vi "FL compute rule weights.vi"(7 "max num consequent membership fcns":i32, 8 "rule-invoked array":bool[](array[boolean]), 9 "output membership factors (u)":dbl[][](array[numeric]), 10 "input membership factors (u)":dbl[][](array[numeric]), 11 "fuzzy system in":T1 {"user MF interpolating polynomials"."coa_x(y) coeff" format="%.4g"; "user MF interpolating polynomials"."Area(y) coeff" format="%.4g"; "user MF interpolating polynomials"."X(y) coeff" format="%.4g"; "user MF interpolating polynomials"."Y(x) coeff" format="%.4g"; "user MF interpolating polynomials"."Y" format="%.4g"; "user MF interpolating polynomials"."X" format="%.4g"; "defuzzification method" items=["Center of Area", "Modified Center of Area", "Center of Sums", "Center of Maximum", "Mean of Maximum"]; "rules"."consequents"."Var Index" min=0; "rules"."consequents"."Cond" items=["=", "!="]; "rules"."consequents"."MF Index" min=0; "rules"."antecedents"."Var Index" min=0; "rules"."antecedents"."Cond" items=["=", "!="]; "rules"."antecedents"."MF Index" min=0; "rules"."consequent implication" items=["Minimum", "Product"]; "rules"."antecedent connective" items=["AND (Minimum)", "AND (Product)", "OR (Maximum)", "OR (Probabilistic)"]; "output variables"."MFs"."shape" items=["Triangle", "Trapezoid", "Singleton", "Sigmoid", "Gaussian", "User-Defined"]; "input variables"."MFs"."shape" items=["Triangle", "Trapezoid", "Singleton", "Sigmoid", "Gaussian", "User-Defined"]}) -> (0 "rule-invoked values?":bool[](array[boolean]), 1 "output membership factors (u)":dbl[][](array[numeric]), 2 "input membership factors (u)":dbl[][](array[numeric]), 3 "fuzzy system out":T1 {"user MF interpolating polynomials"."coa_x(y) coeff" format="%.4g"; "user MF interpolating polynomials"."Area(y) coeff" format="%.4g"; "user MF interpolating polynomials"."X(y) coeff" format="%.4g"; "user MF interpolating polynomials"."Y(x) coeff" format="%.4g"; "user MF interpolating polynomials"."Y" format="%.4g"; "user MF interpolating polynomials"."X" format="%.4g"; "defuzzification method" items=["Center of Area", "Modified Center of Area", "Center of Sums", "Center of Maximum", "Mean of Maximum"]; "rules"."consequents"."Var Index" min=0; "rules"."consequents"."Cond" items=["=", "!="]; "rules"."consequents"."MF Index" min=0; "rules"."antecedents"."Var Index" min=0; "rules"."antecedents"."Cond" items=["=", "!="]; "rules"."antecedents"."MF Index" min=0; "rules"."consequent implication" items=["Minimum", "Product"]; "rules"."antecedent connective" items=["AND (Minimum)", "AND (Product)", "OR (Maximum)", "OR (Probabilistic)"]; "output variables"."MFs"."shape" items=["Triangle", "Trapezoid", "Singleton", "Sigmoid", "Gaussian", "User-Defined"]; "input variables"."MFs"."shape" items=["Triangle", "Trapezoid", "Singleton", "Sigmoid", "Gaussian", "User-Defined"]}, 4 "rule weights":dbl[](array[numeric]))   [LabVIEW 2013, in "NI_Fuzzy_Logic_API.lvlib"]
uses:
  <vilib>/addons/Fuzzy Logic/NI_Fuzzy_Logic_API.lvlib
  <vilib>/addons/Fuzzy Logic/TypeDefs/FL System.ctl
  <vilib>/addons/Fuzzy Logic/TypeDefs/FL Variable.ctl
  <vilib>/addons/Fuzzy Logic/TypeDefs/FL Membership Function.ctl
  <vilib>/addons/Fuzzy Logic/TypeDefs/FL Membership Function Shape.ctl
  <vilib>/addons/Fuzzy Logic/TypeDefs/FL Rule.ctl
  <vilib>/addons/Fuzzy Logic/TypeDefs/FL Antecedent.ctl
  <vilib>/addons/Fuzzy Logic/TypeDefs/FL Modifier.ctl
  <vilib>/addons/Fuzzy Logic/TypeDefs/FL Antecedent Connective.ctl
  <vilib>/addons/Fuzzy Logic/TypeDefs/FL Consequent.ctl
  <vilib>/addons/Fuzzy Logic/TypeDefs/FL Consequent Implication.ctl
  <vilib>/addons/Fuzzy Logic/TypeDefs/FL Defuzzification.ctl
  <vilib>/addons/Fuzzy Logic/TypeDefs/FL Interpolating polynomials.ctl
panel:
  # "IF"
  # "THEN"
  # "IF"
  # "THEN"
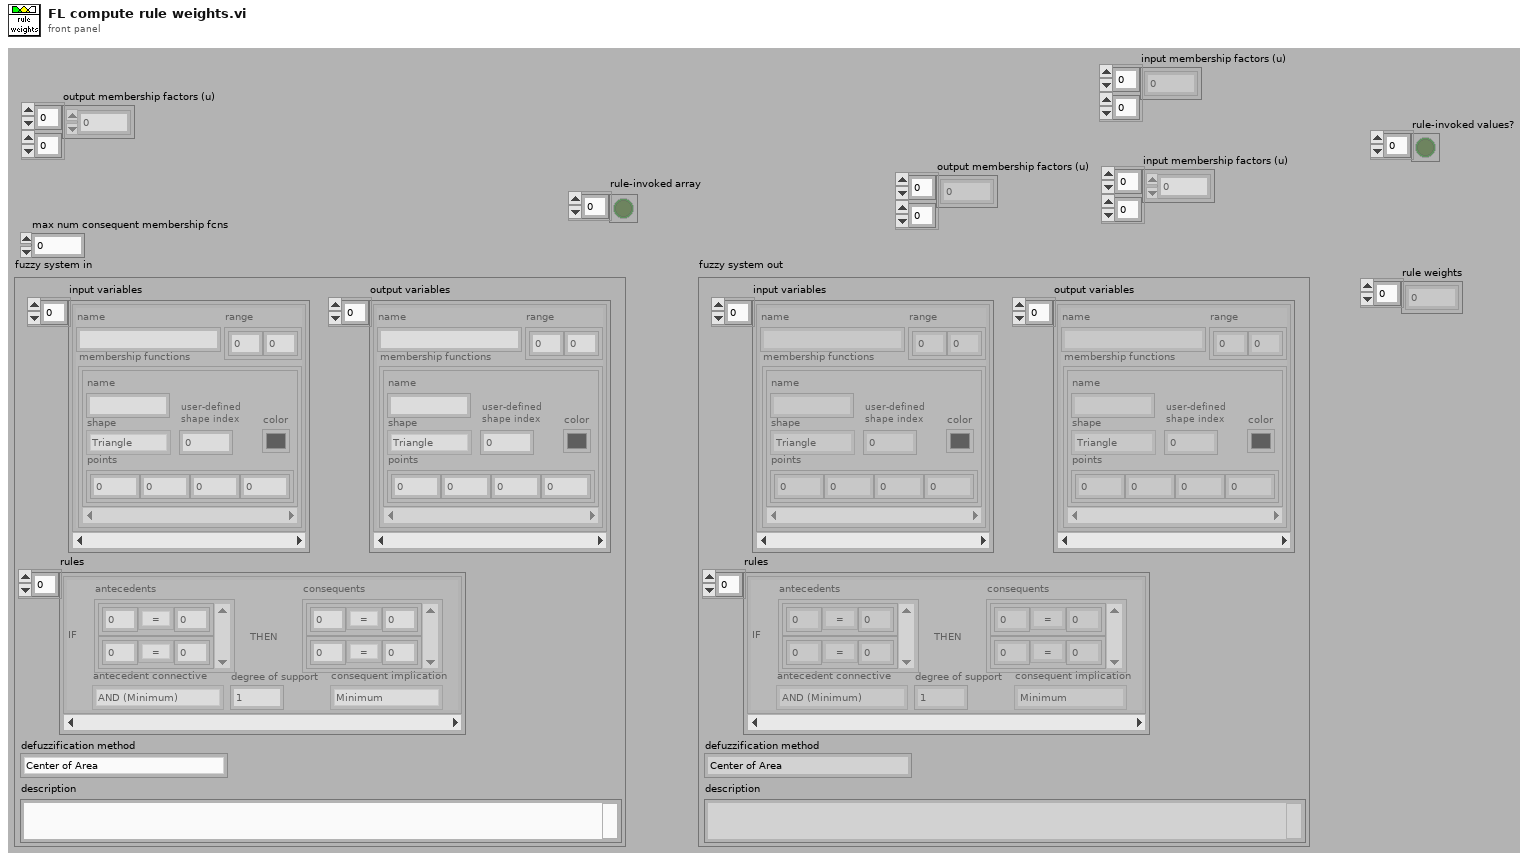
[diagram p1: front panel]
types:
  T1 = typedef "NI_Fuzzy_Logic_API.lvlib/FL System.ctl" = cluster{"input variables":T2[], "output variables":T2[], "rules":T5[], "defuzzification method":T11, "description":string, "user MF interpolating polynomials":T12[]}
  T2 = typedef "NI_Fuzzy_Logic_API.lvlib/FL Variable.ctl" = cluster{"name":string, "range":dbl[], "MFs":T3[]}
  T3 = typedef "NI_Fuzzy_Logic_API.lvlib/FL Membership Function.ctl" = cluster{"name":string, "shape":T4, "points":dbl[], "color":u32, "user-defined shape index":i32}
  T4 = typedef "NI_Fuzzy_Logic_API.lvlib/FL Membership Function Shape.ctl" = u16
  T5 = typedef "NI_Fuzzy_Logic_API.lvlib/FL Rule.ctl" = cluster{"antecedents":T6[], "antecedent connective":T8, "consequents":T9[], "consequent implication":T10, "degree of support":dbl}
  T6 = typedef "NI_Fuzzy_Logic_API.lvlib/FL Antecedent.ctl" = cluster{"Var Index":i32, "MF Index":i32, "Cond":T7}
  T7 = typedef "NI_Fuzzy_Logic_API.lvlib/FL Modifier.ctl" = u16
  T8 = typedef "NI_Fuzzy_Logic_API.lvlib/FL Antecedent Connective.ctl" = u16
  T9 = typedef "NI_Fuzzy_Logic_API.lvlib/FL Consequent.ctl" = cluster{"Var Index":i32, "MF Index":i32, "Cond":T7}
  T10 = typedef "NI_Fuzzy_Logic_API.lvlib/FL Consequent Implication.ctl" = u16
  T11 = typedef "NI_Fuzzy_Logic_API.lvlib/FL Defuzzification.ctl" = u16
  T12 = typedef "NI_Fuzzy_Logic_API.lvlib/FL Interpolating polynomials.ctl" = cluster{"X":dbl[], "Y":dbl[], "Y(x) coeff":dbl[][], "X(y) coeff":dbl[][], "Area(y) coeff":dbl[][], "coa_x(y) coeff":dbl[][]}
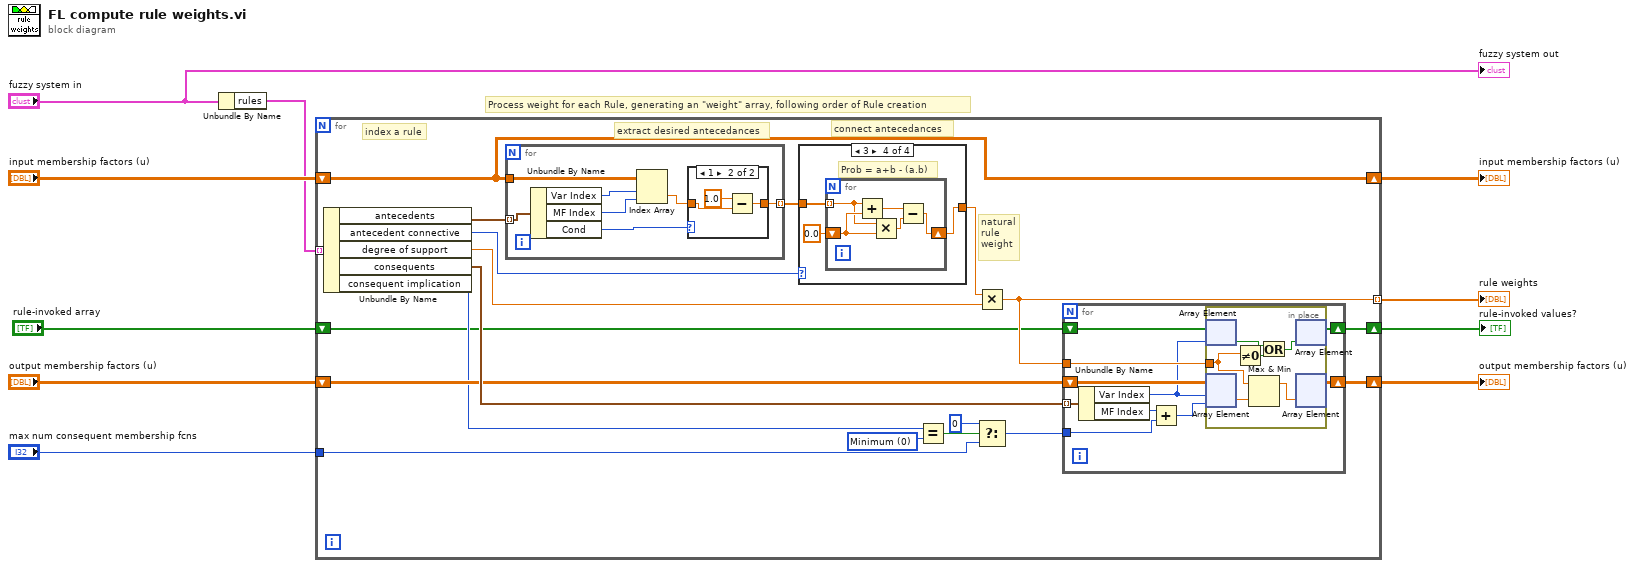
[diagram p0: block diagram]
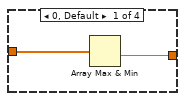
[diagram p2: hidden frame]
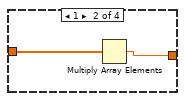
[diagram p3: hidden frame]
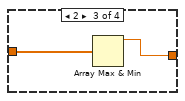
[diagram p4: hidden frame]
diagram:
  # "Process weight for each Rule, generating an \"weight\" array, following order of Rule creation"
  n1 = Unbundle By Name("fuzzy system in") -> ("rules"=w5:T5[])
  n2 = for {
    tunnel: w5 -> [w26] mode=indexing
    tunnel: [w21] -> w10 mode=indexing
    shift-right: [w20] -> w8
    shift-left: "output membership factors (u)" -> [w22]
    shift-right: [w19] -> w6
    shift-left: "input membership factors (u)" -> [w19]
    tunnel: "max num consequent membership fcns" -> [w14]
    shift-right: [w11] -> w1
    shift-left: "rule-invoked array" -> [w12]
    w13 = T10 0 items=["Minimum", "Product"] ("Implication")
    # "natural\nrule\nweight"
    # "extract desired antecedances"
    # "connect antecedances"
    # "index a rule"
    n3 = Unbundle By Name(w26) -> ("antecedents"=w29:T6[], "antecedent connective"=w28:T8, "degree of support"=w24:dbl, "consequents"=w23:T9[], "consequent implication"=w18:T10)
    n4 = for {
      tunnel: w19 -> [w66]
      tunnel: w29 -> [w63] mode=indexing
      tunnel: [w64] -> w27 mode=indexing
      n5 = Unbundle By Name(w63) -> ("Var Index"=w62:i32, "MF Index"=w61:i32, "Cond"=w60:T7)
      n6 = Index Array(array=w66, index (row)=w62, index (col)=w61) -> (element=w65:dbl)
      n7 = case shown="1" w60 {
        tunnel: w65 -> [w67 w69]
        tunnel: [w67 w70] -> w64
        frame 0, Default {
        }
        frame 1 {
          n8 = Subtract(x=1.0, y=w69) -> (x-y=w70:dbl)
        }
      }
    }
    n9 = case shown="3" w28 {
      tunnel: w27 -> [w47 w49 w51 w54]
      tunnel: [w46 w48 w50 w52] -> w25
      frame 0, Default {
        n10 = Array Max & Min(array=w47) -> (min value=w46:dbl)  [unwired: 3 out]
      }
      frame 1 {
        n11 = Multiply Array Elements(1:w49) -> (0:w48:dbl)
      }
      frame 2 {
        n12 = Array Max & Min(array=w51) -> (max value=w50:dbl)  [unwired: 3 out]
      }
      frame 3 {
        # "Prob = a+b - (a.b)"
        n13 = for {
          tunnel: w54 -> [w55] mode=indexing
          shift-right: [w57] -> w52
          shift-left: 0.0 ("Membership") -> [w56]
          n14 = Add(x=w55, y=w56) -> (x+y=w58:dbl)
          n15 = Multiply(x=w55, y=w56) -> (x*y=w59:dbl)
          n16 = Subtract(x=w58, y=w59) -> (x-y=w57:dbl)
        }
      }
    }
    n17 = Equal?(x=w18, y=w13) -> (x = y?=w17:bool)
    n18 = Multiply(x=w25, y=w24) -> (x*y=w21:dbl)
    n19 = Select(t=0, s=w17, f=w14) -> (s? t:f=w15:i32)
    n20 = for {
      tunnel: w23 -> [w39] mode=indexing
      shift-right: [w36] -> w20
      shift-left: w22 -> [w37]
      tunnel: w21 -> [w38]
      tunnel: w15 -> [w35]
      shift-right: [w30] -> w11
      shift-left: w12 -> [w32]
      n21 = Unbundle By Name(w39) -> ("Var Index"=w31:i32, "MF Index"=w34:i32)
      n22 = Add(x=w34, y=w35) -> (x+y=w33:i32)
      n23 = in-place {
        in-place-border: w38 -> [w43]
        n24 = in-place-array #1(w32, w31) -> (w41:bool)
        n25 = in-place-array #2(w37, w31, w33) -> (w45:dbl)
        n26 = Not Equal To 0?(x=w43) -> (x != 0?=w42:bool)
        n27 = Max & Min(x=w43, y=w45) -> (max(x,y)=w44:dbl)  [unwired: 1 out]
        n28 = Or(x=w41, y=w42) -> (x .or. y?=w40:bool)
        n29 = in-place-array #1(w40) -> (w30:bool[])  [unwired: 1 out]
        n30 = in-place-array #2(w44) -> (w36:dbl[][])  [unwired: 2 out]
      }
    }
  }
  "rule weights" <- w10
  "input membership factors (u)" <- w6
  "output membership factors (u)" <- w8
  "rule-invoked values?" <- w1
  "fuzzy system out" <- "fuzzy system in"
